vi "Stop Stage.vi"(8 "error in (no error)":errorcluster, 11 "Stage Actor.lvlib:Stage.lvclass":refnum<class "Stage.lvclass">) -> (0 "error out":errorcluster, 3 "Actor out":refnum<class "Actor.lvclass">)   [LabVIEW 2018, in "Stage Actor.lvlib" / "Stage.lvclass"]
uses:
  Stage.lvclass
  <vilib>/ActorFramework/Actor/Actor.lvclass
  C:/Program Files (x86)/National Instruments/LabVIEW 2018/vi.lib/ActorFramework/Actor/Actor.lvclass
  Stage.lvclass/Stage.ctl
  <instrlib>/Zaber A Series/Zaber A Series.lvlib
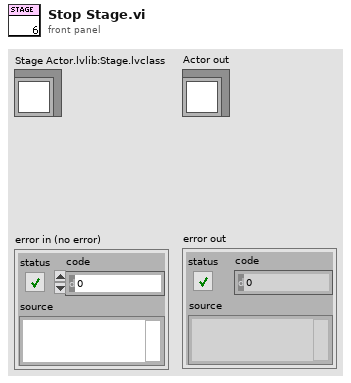
[diagram p1: front panel]
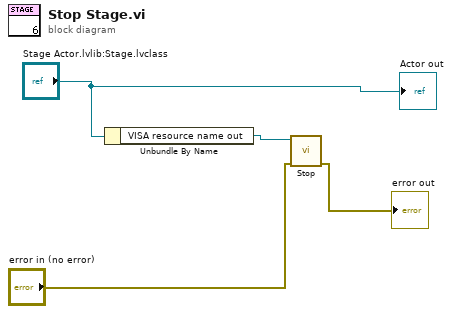
[diagram p0: block diagram]
diagram:
  n1 = Unbundle By Name("Stage Actor.lvlib:Stage.lvclass") -> ("VISA resource name out"=w3:refnum<visa-resource-name>)
  n2 = call <instrlib>:"Stop.vi"("error in (no error)"="error in (no error)", "VISA resource name"=w3) -> ("error out"=→"error out":errorcluster)  [unwired: 8 in, 1 out]
  "Actor out" <- "Stage Actor.lvlib:Stage.lvclass"
